vi "GetVoltageRef.vi"(8 "error in (no error)":errorcluster, 9 "lsecon":T1={"NoiseVariance"=0.001, "IEEESystem"=5, "PMULocations"=[1], "Vindex"=0, "Iindex"=3, "DynamicRef"=""}, 10 "SystemVoltagesRef":cdb[][](array[numeric])) -> (0 "error out":errorcluster, 2 "SystemVoltagesRef Out":cdb[][](array[numeric]))   [LabVIEW 2017, in "AppPlugins.lvlib" / "LSEPlugin.lvclass"]
uses:
  LSEPlugin.lvclass
  Typedefs/LSEConfig.ctl
  Framework/Config_class/Config.lvclass/Config.ctl
  Framework/Config_class/Accessors/Read PARTF Root Directory.vi
  <vilib>/Utility/error.llb/Error Cluster From Error Code.vi
  <vilib>/Utility/file.llb/Read From Spreadsheet File (string).vi
  <vilib>/ErrorRing/Error Ring.xnode
  Visualization/VisualizeApp_class/VisualizeAppLSE.lvclass
  Framework/Config_class/Config.lvclass
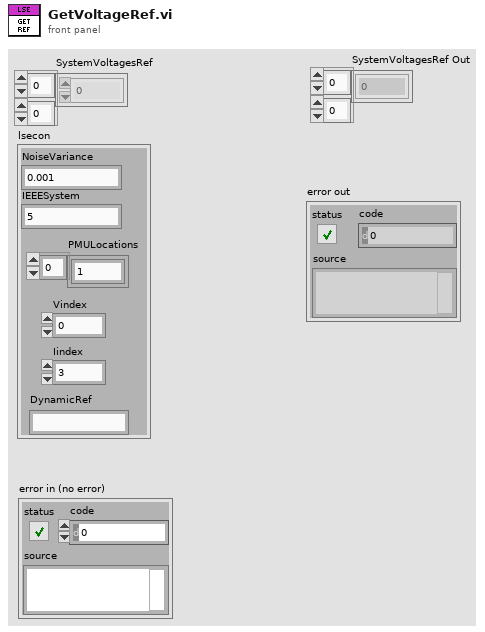
[diagram p1: front panel]
types:
  T1 = typedef "AppPlugins.lvlib/LSEPlugin.lvclass/LSEConfig.ctl" = cluster{"NoiseVariance":dbl, "IEEESystem":u32, "PMULocations":u32[], "Vindex":i32, "Iindex":i32, "DynamicRef":string}
  T2 = typedef "Framework.lvlib/Config.lvclass/RootDir.ctl" = cluster{"pathRootDir":path, "btnOutPath":bool, "OutDir":string, "btnOpenOutputDir":bool, "ScriptDir":string, "btnOpenScriptDir":bool, "TestDir":string, "btnOpenTestDir":bool}
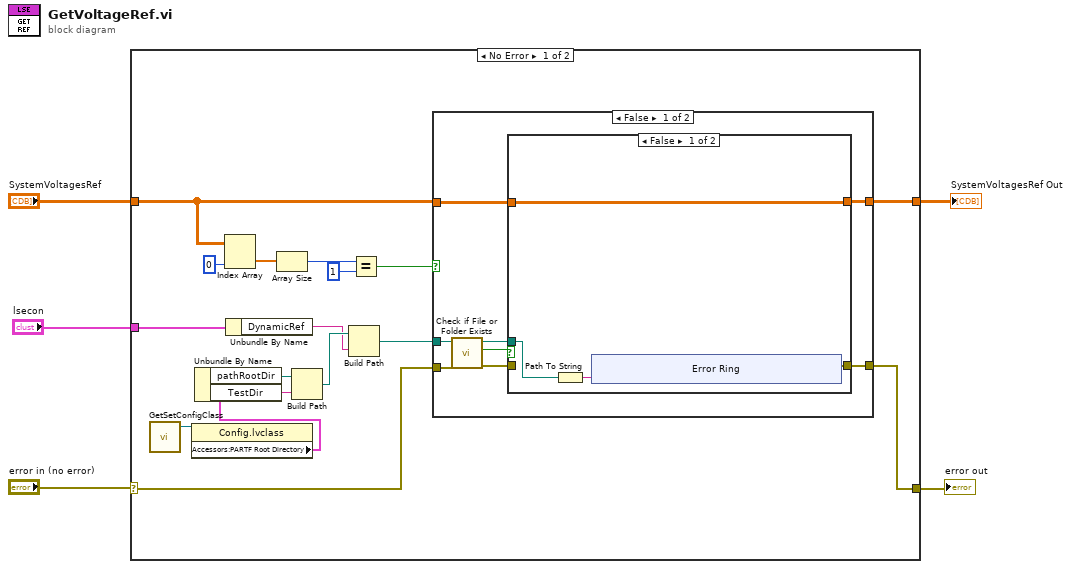
[diagram p0: block diagram]
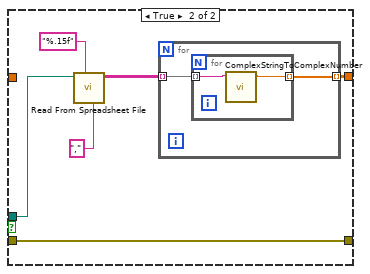
[diagram p2: hidden frame]
diagram:
  n1 = case shown="No Error" "error in (no error)" {
    selector: "error in (no error)" -> [w8 w54]
    tunnel: [w22 w55] -> w5
    tunnel: "SystemVoltagesRef" -> [w18 w55]
    tunnel: "lsecon" -> [w15 _]
    tunnel: [w6 w54] -> w1
    frame No Error {
      n2 = call "GetSetConfigClass.vi"() -> ("Ref out"=w14:refnum<class "Config.lvclass">)  [unwired: 11 in]
      n3 = property class="Config.lvclass"(reference=w14) -> ("Accessors:PARTF Root Directory"=w13:T2)  [unwired: 1 in, 2 out]
      n4 = Unbundle By Name(w13) -> ("pathRootDir"=w12:path, "TestDir"=w11:string)
      n5 = Index Array(array=w18, index (col)=0 ("disabled index (col)")) -> (element=w16:cdb[])  [unwired: 1 in]
      n6 = Unbundle By Name(w15) -> ("DynamicRef"=w9:string)
      n7 = Array Size(array=w16) -> (size(s)=w21:i32)
      n8 = Build Path(base path=w12, name or relative path=w11) -> (appended path=w10:path)
      n9 = Build Path(base path=w10, name or relative path=w9) -> (appended path=w7:path)
      n10 = Equal?(x=w21, y=1) -> (x = y?=w19:bool)
      n11 = case shown="False" w19 {
        tunnel: [w30 w53] -> w22
        tunnel: w18 -> [w23 w53]
        tunnel: w8 -> [w29 w52]
        tunnel: w7 -> [w28 _]
        tunnel: [w24 w52] -> w6
        frame False {
          n12 = call <vilib>:"Check if File or Folder Exists.vi"("error in (no error)"=w29, "path"=w28) -> ("error out"=w25:errorcluster, "file or folder exists?"=w26:bool, "dup path"=w27:path)  [unwired: 7 in]
          n13 = case shown="False" w26 {
            tunnel: [w33 w44] -> w30
            tunnel: w27 -> [w31 w43]
            tunnel: w25 -> [_ w42]
            tunnel: [w34 w42] -> w24
            tunnel: w23 -> [w33 _]
            frame False {
              n14 = Path To String(path=w31) -> (string=w32:string)
              n15 = xnode "Error Ring"("parameter 0"=w32) -> ("error out"=w34:errorcluster)
            }
            frame True {
              n16 = call-poly <vilib>:"Read From Spreadsheet File.vi"("delimiter (\\t)"="," ("delimiter (\\t)"), "format (%s)"="%.15f" ("format (%.3f)"), "file path (dialog if empty)"=w43) -> ("all rows"=w45:string[][])  [unwired: 4 in, 4 out]
              n17 = for {
                tunnel: w45 -> [w49] mode=indexing
                tunnel: [w48] -> w44 mode=indexing
                n18 = for {
                  tunnel: w49 -> [w51] mode=indexing
                  tunnel: [w50] -> w48 mode=indexing
                  n19 = call "ComplexStringToComplexNumber.vi"("String"=w51) -> ("Numeric"=w50:cdb)  [unwired: 10 in]
                }
              }
            }
          }
        }
        frame True {
        }
      }
    }
    frame Error {
    }
  }
  "error out" <- w1
  "SystemVoltagesRef Out" <- w5
